vi "MyFPGA DIO 8-bit Bank.vi"(1 "DIO 7:0 Refnum":refnum<k21>, 2 "OUT 7:0":u8 format="%08b", 3 "DIR 7:0":u8 format="%08b") -> (0 "IN 7:0":u8 format="%08d")   [LabVIEW 2019]
doc: "This VI reads a U8 data bank from or writes the data bank to the specified FPGA I/O item according to the direction of the data flow (<b>DIR 7:0</b>).\nFor each bit of <b>DIR 7:0</b>:\n- DIR: 1 - Write data to the corresponding bit of <b>OUT 7:0</b>\n- DIR: 0 - Read data from the corresponding bit of <b>IN 7:0</b>"
uses:
  <vilib>/rvi/eio/common/nirviEmuTemplateMethod_errors.vi
  <vilib>/eio/EIOMethodNode/EIOMethodNode.xnode
  <vilib>/eio/EIONode/EIONode.xnode
panel:
  # "This VI reads a U8 data bank from or writes the data bank to the specified FPGA I/O item according to the direction of the data flow (DIR 7:0).\nFor each bit of DIR 7:0:\n- DIR: 1 - Write data to the corresponding bit of OUT 7:0\n- DIR: 0 - Read data from the corresponding bit of IN 7:0"
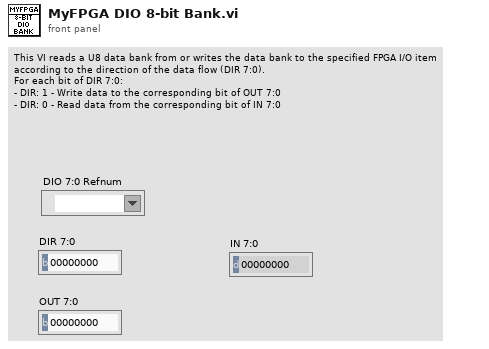
[diagram p1: front panel]
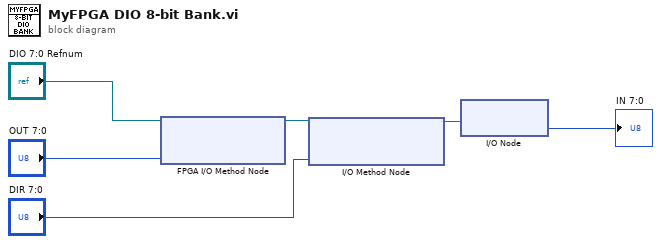
[diagram p0: block diagram]
diagram:
  n1 = xnode "FPGA I/O Method Node"("FPGA I/O In"="DIO 7:0 Refnum", "Data"="OUT 7:0") -> ("FPGA I/O Out"=w4:refnum<k21>)
  n2 = xnode "I/O Method Node"("FPGA I/O In"=w4, "Enable"="DIR 7:0") -> ("FPGA I/O Out"=w5:refnum<k21>)
  n3 = xnode "I/O Node"("FPGA I/O In"=w5) -> ("I/O Item"=→"IN 7:0":u8)  [unwired: 1 out]
